vi "AutoDrive.vi"(5 "Motor Duration (s)":dbl=1.0 caption="Time Target (s)", 7 "Direction":enum16{"Forwards", "Backwards", "Left", "Right"}(ring), 8 "error in (no error)":errorcluster, 11 "RobotDriveDevRef":T1={"DevStatus"={"status"=FALSE, "code"=0, "source"=""}, "Motors[]"=[], "Square Inputs"=FALSE, "Max Output"=1.0}) -> (0 "error out":errorcluster, 3 "RobotDriveDevRefOut":T1={"DevStatus"={"status"=FALSE, "code"=0, "source"=""}, "Motors[]"=[], "Square Inputs"=FALSE, "Max Output"=1.0})   [LabVIEW 2015]
uses:
  <vilib>/Rock Robotics/WPI/RobotDrive/WPI_RobotDriveDevRef.ctl
  <vilib>/Rock Robotics/WPI/MotorControl/WPI_MotorControlDeviceRef.ctl
  <vilib>/Rock Robotics/SystemInterfaces/Typedef/FPGA_TypedefDigitalModule.ctl
  <vilib>/Rock Robotics/SystemInterfaces/DIO/FPGA_DIOPWMChannel.ctl
  <vilib>/Rock Robotics/WPI/PWM/WPI_PWMDeadband.ctl
  <vilib>/Rock Robotics/WPI/CAN/Jaguar/SubVIs/WPI_CANJaguar_ControlMode.ctl
  <vilib>/Rock Robotics/WPI/PWM/WPI_PWMTransform_ConPane.ctl
  <vilib>/Rock Robotics/WPI/RobotDrive/WPI_RobotDriveMecanumDrive_Cartesian.vi
panel:
  in  "DriveZ":dbl
  in  "DriveY":dbl
  in  "DriveX":dbl
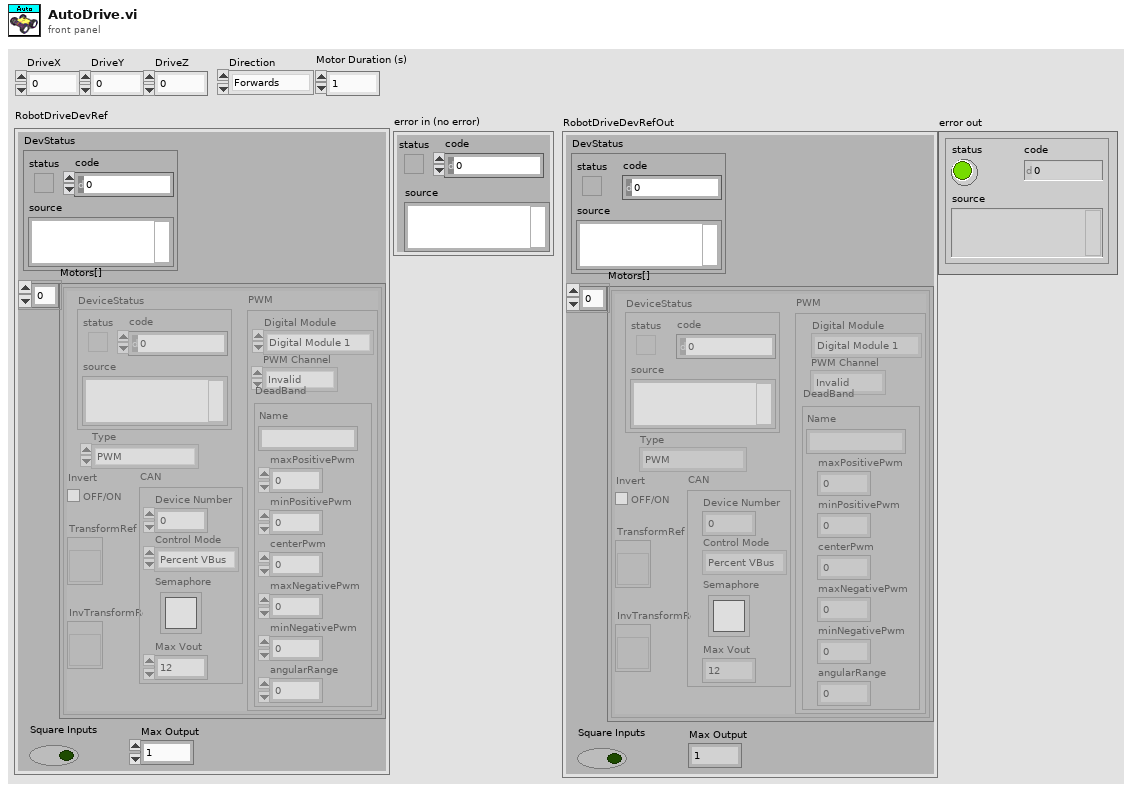
[diagram p1: front panel]
types:
  T1 = typedef "WPI_RobotDriveDevRef.ctl" = cluster{"DevStatus":errorcluster, "Motors[]":T2[], "Square Inputs":bool, "Max Output":dbl}
  T2 = typedef "WPI_MotorControlDeviceRef.ctl" = cluster{"DeviceStatus":errorcluster, "Type":enum16{"PWM", "CAN"}, "PWM":cluster{"Digital Module":T3, "PWM Channel":T4, "DeadBand":T5}, "CAN":cluster{"Device Number":u8, "Control Mode":T6, "Semaphore":T7, "Max Vout":dbl}, "Invert":bool, "TransformRef":T8, "InvTransformRef":T8}
  T3 = typedef "FPGA_TypedefDigitalModule.ctl" = enum16{"Digital Module 1", "Digital Module 2"}
  T4 = typedef "FPGA_DIOPWMChannel.ctl" = enum8{"PWM 1", "PWM 2", "PWM 3", "PWM 4", "PWM 5", "PWM 6", "PWM 7", "PWM 8", "PWM 9", "PWM 10", "Invalid"}
  T5 = typedef "WPI_PWMDeadband.ctl" = cluster{"Name":string, "maxPositivePwm":i32, "minPositivePwm":i32, "centerPwm":i32, "maxNegativePwm":i32, "minNegativePwm":i32, "angularRange":u16}
  T6 = typedef "WPI_CANJaguar_ControlMode.ctl" = enum8{"Percent VBus", "Current", "Speed", "Position", "Voltage"}
  T7 = typedef "Semaphore RefNum" = refnum<k1>
  T8 = typedef "WPI_PWMTransform_ConPane.ctl" = refnum<vi>
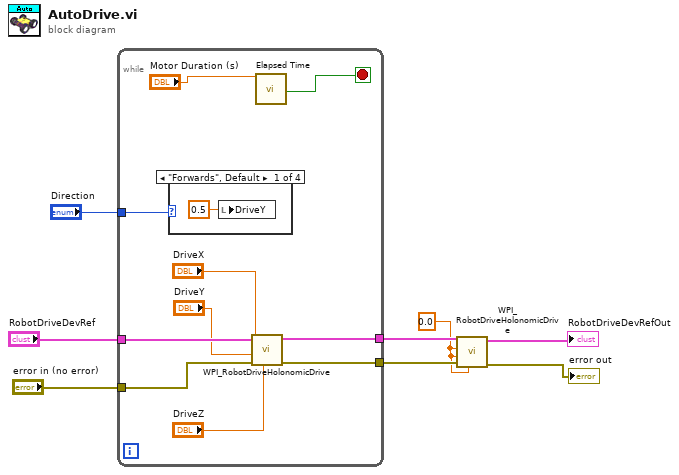
[diagram p0: block diagram]
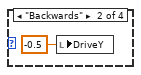
[diagram p2: hidden frame]
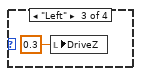
[diagram p3: hidden frame]
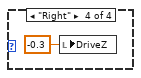
[diagram p4: hidden frame]
diagram:
  w3 = 0.0 ("X")
  n1 = while {
    tunnel: "RobotDriveDevRef" -> [w18]
    tunnel: "error in (no error)" -> [w17]
    tunnel: [w14] -> w5
    tunnel: [w13] -> w4
    tunnel: "Direction" -> [w9]
    stop <- w16 stop-if-true
    n2 = case shown="\"Forwards\", Default" w9 {
      frame "Forwards", Default {
        n3 = local write "DriveY"(0.5 ("DriveY")) -> ()
      }
      frame "Backwards" {
        n4 = local write "DriveY"(-0.5 ("DriveY")) -> ()
      }
      frame "Left" {
        n5 = local write "DriveZ"(0.3 ("DriveZ")) -> ()
      }
      frame "Right" {
        n6 = local write "DriveZ"(-0.3 ("DriveZ")) -> ()
      }
    }
    n7 = call-poly <vilib>:"WPI_RobotDriveHolonomicDrive.vi"("Rotation"="DriveZ", "error in (no error)"=w17, "Y"="DriveY", "X"="DriveX", "RobotDriveDevRef"=w18) -> ("error out"=w13:errorcluster, "RobotDriveDevRef"=w14:T1)  [unwired: 4 in, 1 out]
    n8 = call "Elapsed Time"("Time Target (s)"="Motor Duration (s)") -> ("Time has Elapsed"=w16:bool)  [unwired: 11 in, 7 out]
  }
  n9 = call-poly <vilib>:"WPI_RobotDriveHolonomicDrive.vi"("Rotation"=w3, "error in (no error)"=w4, "Y"=w3, "X"=w3, "RobotDriveDevRef"=w5) -> ("error out"=→"error out":errorcluster, "RobotDriveDevRef"=→"RobotDriveDevRefOut":T1)  [unwired: 4 in, 1 out]
